vi "Add Array Data Channels.vi"(8 "error in (no error)":errorcluster, 10 "array elements":T2[](array[typedef]), 11 "section refnum in":T1 format="%.0x") -> (0 "error out":errorcluster, 2 "channel refs":T1[](array[typedef]) format="%.0x", 3 "array refnum":T1 format="%.0x")   [LabVIEW 2020, in "Instrument Addon Scripting API.lvlib"]
doc: "Adds channels under the Data Array section provided as reference input."
uses:
  Instrument Addon Scripting API.lvlib
  <vilib>/NI VeriStand/Custom Device API/Custom Device Item Ref.ctl
  TypeDefs/Array Element.ctl
  <vilib>/NI VeriStand/Custom Device API/Custom Device Channel.ctl
  <vilib>/NI VeriStand/Custom Device API/Custom Device Channel Type.ctl
  Shared Directory/Constants.vi
  <vilib>/NI VeriStand/Custom Device API/Custom Device API.lvlib
  Shared Directory/Instrument Addon Shared.lvlib
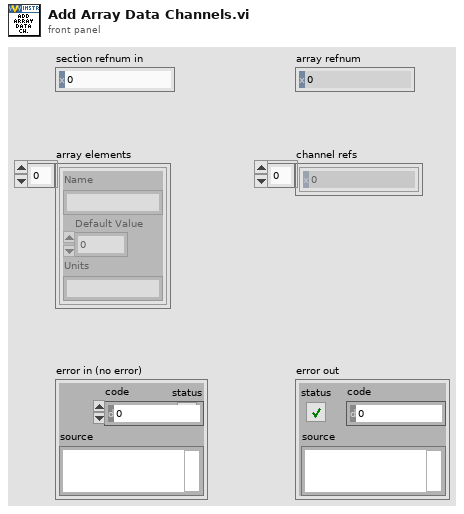
[diagram p1: front panel]
types:
  T1 = typedef "Custom Device API.lvlib/Custom Device Item Ref.ctl" = u64
  T2 = typedef "Instrument Addon Scripting API.lvlib/Array Element.ctl" = cluster{"Name":string, "Default Value":dbl, "Units":string}
  T3 = typedef "Custom Device API.lvlib/Custom Device Channel.ctl" = cluster{"Type":T4, "Units":string, "Default Value":dbl, "Faultable":bool, "Scalable":bool}
  T4 = typedef "Custom Device API.lvlib/Custom Device Channel Type.ctl" = enum16{"Input", "Output"}
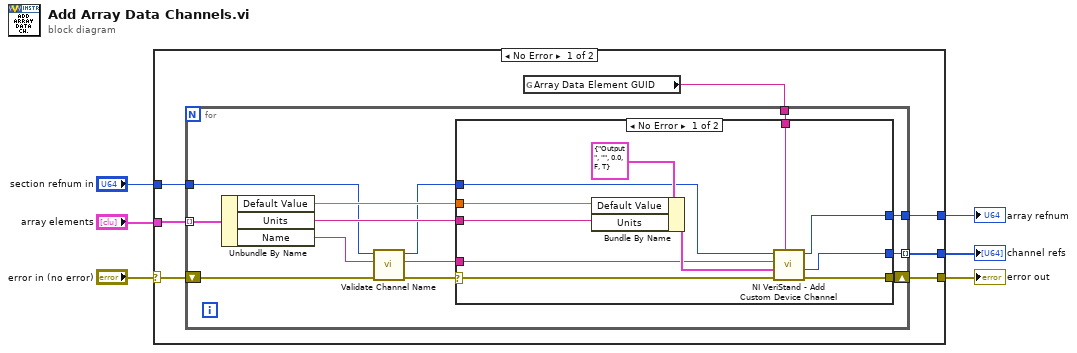
[diagram p0: block diagram]
diagram:
  n1 = case shown="No Error" "error in (no error)" {
    selector: "error in (no error)" -> [w10 w41]
    tunnel: [w13 w41] -> w6
    tunnel: "section refnum in" -> [w12 w40]
    tunnel: "array elements" -> [w8 _]
    tunnel: [w9 _] -> w2
    tunnel: [w7 w40] -> w1
    frame No Error {
      n2 = global read "Constants.vi" "Array Data Element GUID"() -> (w11:string)
      n3 = for {
        shift-right: [w26] -> w13
        shift-left: w10 -> [w16]
        tunnel: w11 -> [w25]
        tunnel: w12 -> [w14]
        tunnel: w8 -> [w24] mode=indexing
        tunnel: [w21] -> w9 mode=indexing
        tunnel: [w20] -> w7
        n4 = Unbundle By Name(w24) -> ("Default Value"=w23:dbl, "Units"=w22:string, "Name"=w15:string)
        n5 = call "Validate Channel Name.vi"("error in (no error)"=w16, "Name In"=w15, "Refnum In"=w14) -> ("error out"=w17:errorcluster, "Name Out"=w18:string, "Refnum Out"=w19:T1)  [unwired: 6 in]
        n6 = case shown="No Error" w17 {
          selector: w17 -> [w29 w39]
          tunnel: [w37 w39] -> w26
          tunnel: w25 -> [w34 _]
          tunnel: w19 -> [w33 w38]
          tunnel: w23 -> [w32 _]
          tunnel: w22 -> [w31 _]
          tunnel: w18 -> [w30 _]
          tunnel: [w28 _] -> w21
          tunnel: [w27 w38] -> w20
          frame No Error {
            n7 = Bundle By Name(cluster=T3 {"Type"=enum."Output", "Units"="", "Default Value"=0.0, "Faultable"=FALSE, "Scalable"=TRUE} ("Channel"), "Default Value"=w32, "Units"=w31) -> (w35:T3)
            n8 = call <vilib>:"NI VeriStand - Add Custom Device Channel.vi"("GUID (Default Channel)"=w34, "error in (no error)"=w29, "Channel"=w35, "Channel Name"=w30, "Parent Ref in"=w33) -> ("error out"=w37:errorcluster, "Channel Ref"=w28:T1, "Parent Ref out"=w27:T1)  [unwired: 3 in, 1 out]
          }
          frame Error {
          }
        }
      }
    }
    frame Error {
    }
  }
  "error out" <- w6
  "channel refs" <- w2
  "array refnum" <- w1
